vi "HSMS Notifier Data To String.vi"(8 "error in (no error)":errorcluster, 11 "Notifier Data":T1) -> (0 "error out":errorcluster, 3 "String":string)   [LabVIEW 2020, in "SECS Communication.lvlib" / "HSMS Class.lvclass"]
uses:
  HSMS Class.lvclass
  Notifier Data.ctl
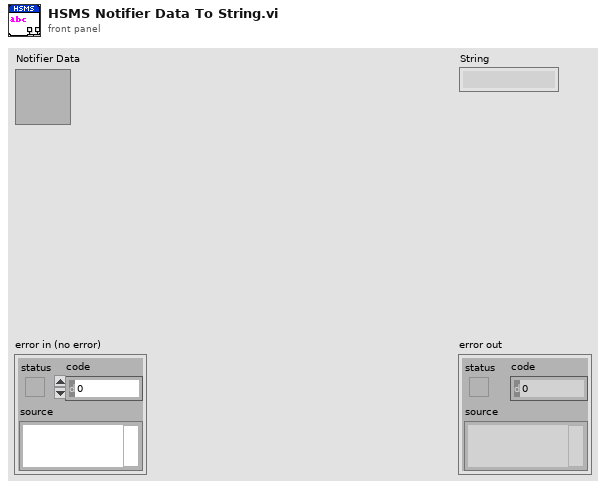
[diagram p1: front panel]
types:
  T1 = typedef "SECS Communication.lvlib/HSMS Class.lvclass/Notifier Data.ctl" = cluster{"Notifier Type":T2, "Data":variant, "Time":timestamp}
  T2 = typedef "SECS Communication.lvlib/HSMS Class.lvclass/Notifier Type.ctl" = enum16{"TCPIP Connect", "TCPIP Disconnect", "Receive Message", "Send Message", "T3 Timeout", "T6 Timeout", "T7 Timeout", "Error", "Stop"}
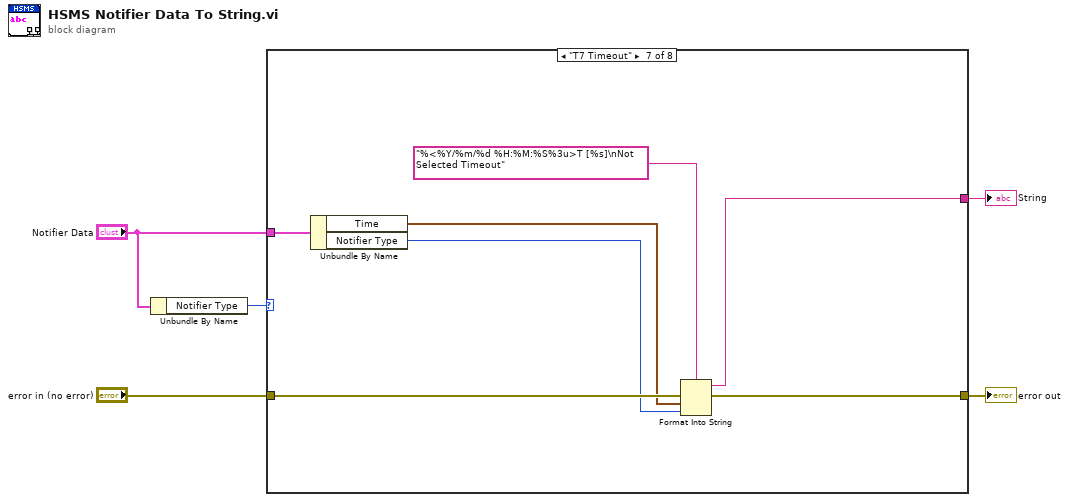
[diagram p0: block diagram]
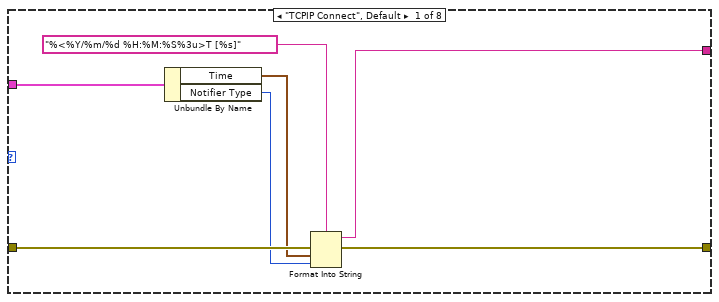
[diagram p2: hidden frame]
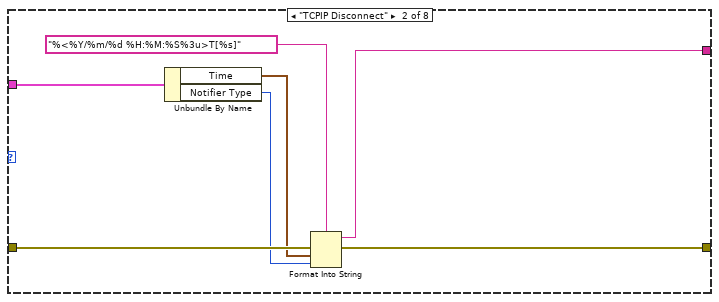
[diagram p3: hidden frame]
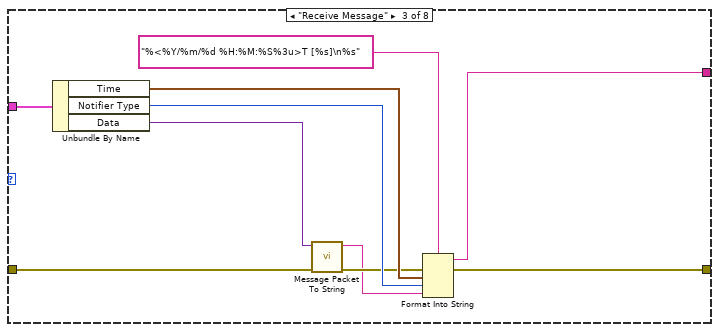
[diagram p4: hidden frame]
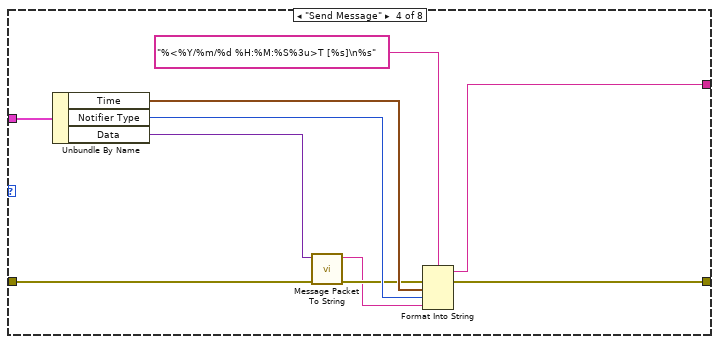
[diagram p5: hidden frame]
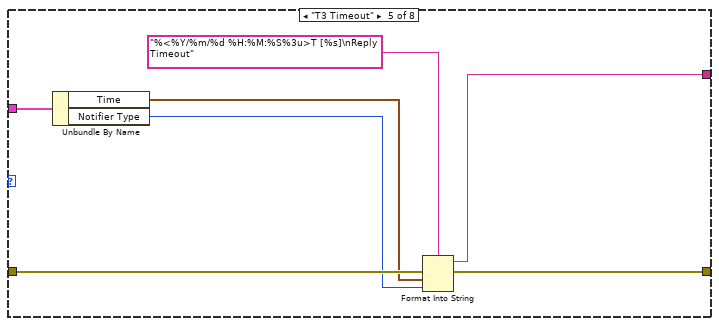
[diagram p6: hidden frame]
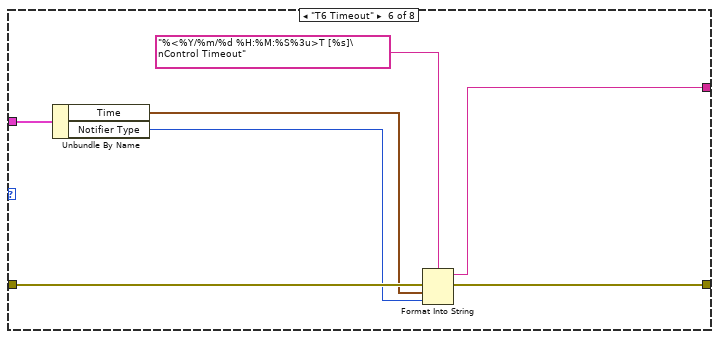
[diagram p7: hidden frame]
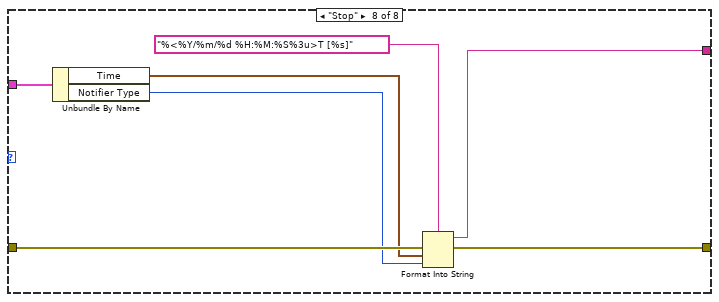
[diagram p8: hidden frame]
diagram:
  n1 = Unbundle By Name("Notifier Data") -> ("Notifier Type"=w4:T2)
  n2 = case shown="\"T7 Timeout\"" w4 {
    tunnel: "error in (no error)" -> [w11 w18 w23 w33 w45 w52 w59 w66]
    tunnel: "Notifier Data" -> [w12 w19 w29 w39 w46 w53 w60 w67]
    tunnel: [w7 w14 w25 w35 w41 w48 w55 w62] -> w2
    tunnel: [w6 w13 w24 w34 w40 w47 w54 w61] -> w1
    frame "TCPIP Connect", Default {
      n3 = Unbundle By Name(w12) -> ("Time"=w10:timestamp, "Notifier Type"=w8:T2)
      n4 = Format Into String(format string="%<%Y/%m/%d %H:%M:%S%3u>T [%s]", error in=w11, w10, w8) -> (resulting string=w6:string, error out=w7:errorcluster)  [unwired: 1 in]
    }
    frame "TCPIP Disconnect" {
      n5 = Unbundle By Name(w19) -> ("Time"=w17:timestamp, "Notifier Type"=w15:T2)
      n6 = Format Into String(format string="%<%Y/%m/%d %H:%M:%S%3u>T[%s]", error in=w18, w17, w15) -> (resulting string=w13:string, error out=w14:errorcluster)  [unwired: 1 in]
    }
    frame "Receive Message" {
      n7 = Unbundle By Name(w29) -> ("Time"=w28:timestamp, "Notifier Type"=w26:T2, "Data"=w22:variant)
      n8 = call "Message Packet To String.vi"("error in (no error)"=w23, "Message Packet"=w22) -> ("error out"=w21:errorcluster, "String"=w20:string)  [unwired: 8 in]
      n9 = Format Into String(format string="%<%Y/%m/%d %H:%M:%S%3u>T [%s]\n%s", error in=w21, w28, w26, w20) -> (resulting string=w24:string, error out=w25:errorcluster)  [unwired: 1 in]
    }
    frame "Send Message" {
      n10 = Unbundle By Name(w39) -> ("Time"=w38:timestamp, "Notifier Type"=w36:T2, "Data"=w32:variant)
      n11 = call "Message Packet To String.vi"("error in (no error)"=w33, "Message Packet"=w32) -> ("error out"=w31:errorcluster, "String"=w30:string)  [unwired: 8 in]
      n12 = Format Into String(format string="%<%Y/%m/%d %H:%M:%S%3u>T [%s]\n%s", error in=w31, w38, w36, w30) -> (resulting string=w34:string, error out=w35:errorcluster)  [unwired: 1 in]
    }
    frame "T3 Timeout" {
      n13 = Unbundle By Name(w46) -> ("Time"=w44:timestamp, "Notifier Type"=w42:T2)
      n14 = Format Into String(format string="%<%Y/%m/%d %H:%M:%S%3u>T [%s]\nReply Timeout", error in=w45, w44, w42) -> (resulting string=w40:string, error out=w41:errorcluster)  [unwired: 1 in]
    }
    frame "T6 Timeout" {
      n15 = Unbundle By Name(w53) -> ("Time"=w51:timestamp, "Notifier Type"=w49:T2)
      n16 = Format Into String(format string="%<%Y/%m/%d %H:%M:%S%3u>T [%s]\nControl Timeout", error in=w52, w51, w49) -> (resulting string=w47:string, error out=w48:errorcluster)  [unwired: 1 in]
    }
    frame "T7 Timeout" {
      n17 = Unbundle By Name(w60) -> ("Time"=w58:timestamp, "Notifier Type"=w56:T2)
      n18 = Format Into String(format string="%<%Y/%m/%d %H:%M:%S%3u>T [%s]\nNot Selected Timeout", error in=w59, w58, w56) -> (resulting string=w54:string, error out=w55:errorcluster)  [unwired: 1 in]
    }
    frame "Stop" {
      n19 = Unbundle By Name(w67) -> ("Time"=w65:timestamp, "Notifier Type"=w63:T2)
      n20 = Format Into String(format string="%<%Y/%m/%d %H:%M:%S%3u>T [%s]", error in=w66, w65, w63) -> (resulting string=w61:string, error out=w62:errorcluster)  [unwired: 1 in]
    }
  }
  "error out" <- w2
  "String" <- w1
